vi "Query Instrument.vi"(8 "error in":errorcluster caption="error out", 11 "VISA resource name (Eingang)":refnum<visa-resource-name>) -> (0 "error out":errorcluster, 1 "Firmware":dbl, 2 "Versionsstring":string, 3 "VISA resource name (Ausgang)":refnum<visa-resource-name>)   [LabVIEW 2018, in "JULABO DeviceDriver.lvlib"]
doc: "This VI identifies the connected unit by the units VERSION string"
uses:
  JULABO DeviceDriver.lvlib
  <vilib>/Utility/error.llb/whitespace.ctl
  InstrumentType.ctl
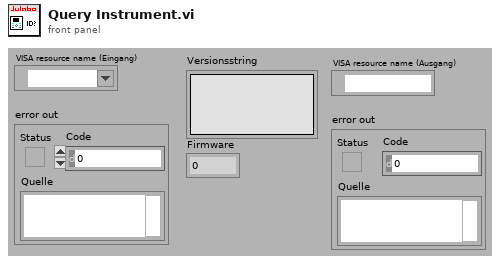
[diagram p1: front panel]
types:
  T1 = typedef "JULABO DeviceDriver.lvlib/InstrumentType.ctl" = enum8{"Default", "FC-Series", "HT30/HT60", "LC4"}
  T2 = typedef "whitespace.ctl" = u16
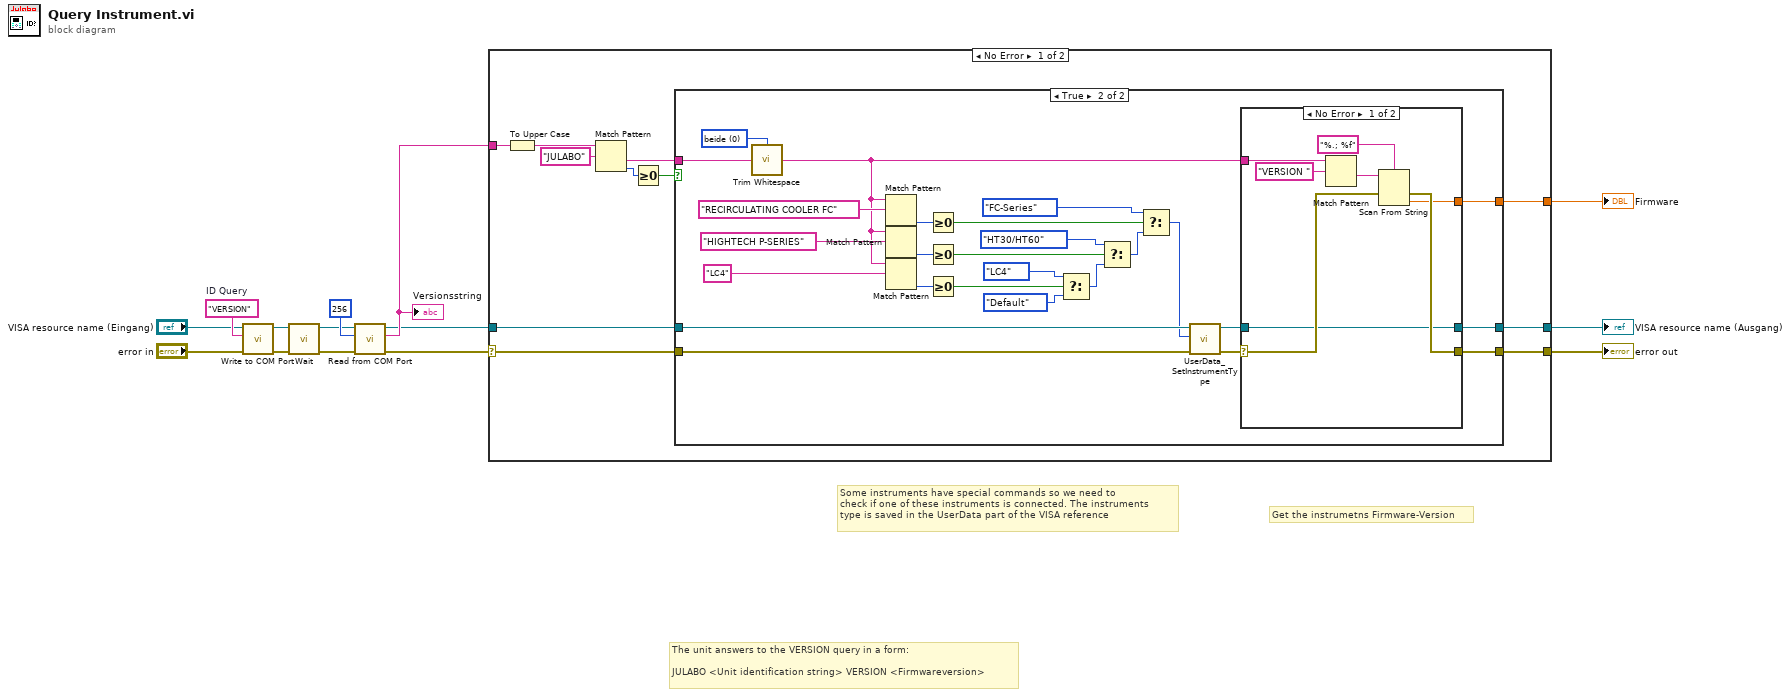
[diagram p0: block diagram]
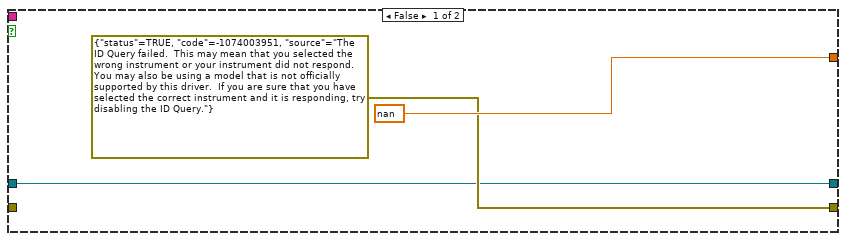
[diagram p2: hidden frame]
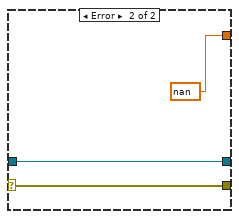
[diagram p3: hidden frame]
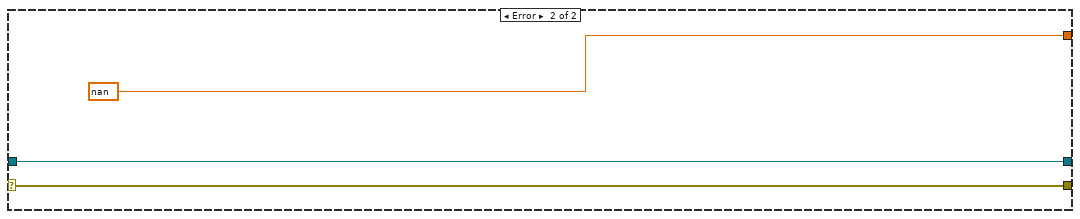
[diagram p4: hidden frame]
diagram:
  w14 = "VERSION"  # ID Query
  # "Get the instrumetns Firmware-Version"
  # "Some instruments have special commands so we need to\ncheck if one of these instruments is connected. The instruments\ntype is saved in the UserData part of the VISA reference"
  # "The unit answers to the VERSION query in a form:\n\nJULABO <Unit identification string> VERSION <Firmwareversion>"
  n1 = call "Write to COM Port.vi"("error in"="error in", "Command (input)"=w14, "VISA resource name in"="VISA resource name (Eingang)") -> ("error out"=w1:errorcluster, "VISA resource name out"=w4:refnum<visa-resource-name>)  [unwired: 7 in]
  n2 = call "Wait.vi"("error in"=w1, "VISA resource name in"=w4) -> ("error out"=w2:errorcluster, "VISA resource name out"=w3:refnum<visa-resource-name>)  [unwired: 4 in]
  n3 = call "Read from COM Port.vi"("error in"=w2, "Byte to Read (-1:All)"=u32 256, "VISA resource name in"=w3) -> ("error out"=w6:errorcluster, "String (output)"=w11:string, "VISA resource name out"=w7:refnum<visa-resource-name>)  [unwired: 5 in, 1 out]
  "Versionsstring" <- w11
  n4 = case shown="No Error" w6 {
    selector: w6 -> [w16 w68]
    tunnel: w11 -> [w25 _]
    tunnel: [w24 w68] -> w10
    tunnel: [w18 nan] -> w9
    tunnel: w7 -> [w17 w66]
    tunnel: [w15 w66] -> w5
    frame No Error {
      n5 = To Upper Case(1:w25) -> (0:w22:string)
      n6 = Match Pattern(string=w22, regular expression="JULABO" ("gültiger Ausdruck")) -> (after substring=w21:string, offset past match=w20:i32)  [unwired: 1 in, 2 out]
      n7 = Greater Or Equal To 0?(x=w20) -> (x >= 0?=w19:bool)
      n8 = case shown="True" w19 {
        tunnel: [errorcluster {"status"=TRUE, "code"=-1074003951, "source"="The ID Query failed.  This may mean that you selected the wrong instrument or your instrument did not respond.  You may also be using a model that is not officially supported by this driver.  If you are sure that you have selected the correct instrument and it is responding, try disabling the ID Query."} ("error out") w54] -> w24
        tunnel: w21 -> [_ w51]
        tunnel: [nan w53] -> w18
        tunnel: w17 -> [w26 w49]
        tunnel: w16 -> [_ w48]
        tunnel: [w26 w46] -> w15
        frame False {
        }
        frame True {
          w52 = T2 0 items=["beide", "Stringanfang", "Stringende"] ("location (both)")
          n9 = call <vilib>:"Trim Whitespace.vi"("string"=w51, "location (both)"=w52) -> ("trimmed string"=w39:string)
          n10 = Match Pattern(string=w39, regular expression="RECIRCULATING COOLER FC") -> (offset past match=w42:i32)  [unwired: 1 in, 3 out]
          n11 = Match Pattern(string=w39, regular expression="HIGHTECH P-SERIES") -> (offset past match=w44:i32)  [unwired: 1 in, 3 out]
          n12 = Match Pattern(string=w39, regular expression="LC4") -> (offset past match=w40:i32)  [unwired: 1 in, 3 out]
          n13 = Greater Or Equal To 0?(x=w42) -> (x >= 0?=w38:bool)
          n14 = Greater Or Equal To 0?(x=w44) -> (x >= 0?=w33:bool)
          n15 = Greater Or Equal To 0?(x=w40) -> (x >= 0?=w37:bool)
          n16 = Select(t=InstrumentType."LC4" ("InstrumentType"), s=w37, f=InstrumentType."Default" ("InstrumentType")) -> (s? t:f=w34:T1)
          n17 = Select(t=InstrumentType."HT30/HT60" ("InstrumentType"), s=w33, f=w34) -> (s? t:f=w30:T1)
          n18 = Select(t=InstrumentType."FC-Series" ("InstrumentType"), s=w38, f=w30) -> (s? t:f=w31:T1)
          n19 = call "UserData_SetInstrumentType.vi"("Fehler (Eingang)"=w48, "InstrumentType"=w31, "VISA resource name in"=w49) -> ("Fehler (Ausgang)"=w47:errorcluster, "VISA resource name out"=w45:refnum<visa-resource-name>)  [unwired: 3 in]
          n20 = case shown="No Error" w47 {
            selector: w47 -> [w56 w65]
            tunnel: w39 -> [w60 _]
            tunnel: [w62 w65] -> w54
            tunnel: [w61 nan] -> w53
            tunnel: [w55 w63] -> w46
            tunnel: w45 -> [w55 w63]
            frame No Error {
              n21 = Match Pattern(string=w60, regular expression="VERSION " ("Format-String")) -> (after substring=w58:string)  [unwired: 1 in, 3 out]
              n22 = Scan From String(format string="%.; %f" ("Format-String"), input string=w58, error in=w56) -> (error out=w62:errorcluster, output 1=w61:dbl)  [unwired: 2 in, 2 out]
            }
            frame Error {
            }
          }
        }
      }
    }
    frame Error {
    }
  }
  "VISA resource name (Ausgang)" <- w5
  "error out" <- w10
  "Firmware" <- w9
